vi "dfd_Lattice AR Normalization (Basic).vi"(7 "scale type":T1, 10 "coefficients k":dbl[](array[numeric]) format="%.2f", 11 "x":dbl[](array[numeric])) -> (2 "norm":dbl[](array[numeric]) format="%.2f", 3 "y":dbl[](array[numeric]))   [LabVIEW 2017, in "NI_DigFilter_FXP.lvlib"]
uses:
  <vilib>/addons/Digital Filter Design/NI_DigFilter_FXP.lvlib
  <vilib>/addons/Digital Filter Design/_Objects.llb/DFD Coef Norm Type.ctl
  <vilib>/addons/Digital Filter Design/NI_DigFilterLicensed.lvlib
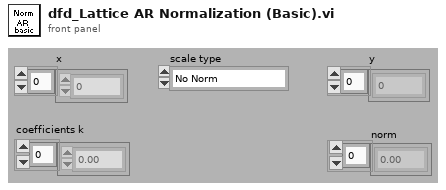
[diagram p1: front panel]
types:
  T1 = typedef "NI_DigFilterLicensed.lvlib/DFD Coef Norm Type.ctl" = enum16{"No Norm", "Time Domain 1-Norm", "Time Domain 2-Norm", "Time Domain Inf-Norm"}
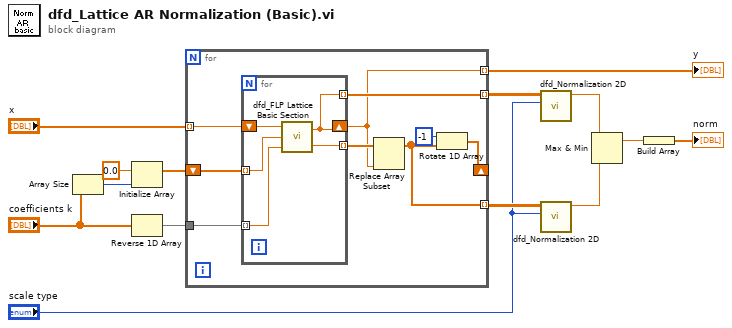
[diagram p0: block diagram]
diagram:
  n1 = Array Size(array="coefficients k") -> (size(s)=w12:i32)
  n2 = Initialize Array(0.0 ("element"), w12) -> (w14:dbl[])
  n3 = Reverse 1D Array(array="coefficients k") -> (reversed array=w11:dbl[])
  n4 = for {
    tunnel: w11 -> [w23]
    shift-right: [w21] -> _
    shift-left: w14 -> [w20]
    tunnel: [w19] -> w6 mode=indexing
    tunnel: [w18] -> w7 mode=indexing
    tunnel: "x" -> [w16] mode=indexing
    tunnel: [w15] -> w1 mode=indexing
    n5 = for {
      shift-right: [w24] -> w15
      shift-left: w16 -> [w28]
      tunnel: w20 -> [w27] mode=indexing
      tunnel: w23 -> [w26] mode=indexing
      tunnel: [w25] -> w22 mode=indexing
      tunnel: [w24] -> w19 mode=indexing
      n6 = call <vilib>:"dfd_FLP Lattice Basic Section.vi"("k(m)"=w26, "w(m-1)"=w27, "x(m)"=w28) -> ("w(m)"=w25:dbl, "x(m-1)"=w24:dbl)
    }
    n7 = Replace Array Subset(array=w22, new element=w15) -> (w18:dbl[])  [unwired: 1 in]
    n8 = Rotate 1D Array(1:w18, 2:-1 ("n")) -> (0:w21:dbl[])
  }
  "y" <- w1
  n9 = call <vilib>:"dfd_Normalization 2D.vi"("scale type"="scale type", "2D Array (col-major)"=w6) -> ("max norm"=w4:dbl)  [unwired: 9 out]
  n10 = call <vilib>:"dfd_Normalization 2D.vi"("scale type"="scale type", "2D Array (col-major)"=w7) -> ("max norm"=w3:dbl)  [unwired: 9 out]
  n11 = Max & Min(x=w4, y=w3) -> (max(x,y)=w2:dbl)  [unwired: 1 out]
  n12 = Build Array(w2) -> (→"norm":dbl[])
